vi "ImageDQStagePosition.vi"(11 "Image in":refnum<class "Image.lvclass">) -> (3 "Image out":refnum<class "Image.lvclass">)   [LabVIEW 2012, in "Image.lvclass"]
uses:
  classes/Image.lvclass
  classes/Image.lvclass/Image.ctl
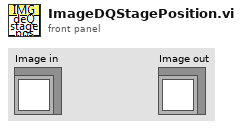
[diagram p1: front panel]
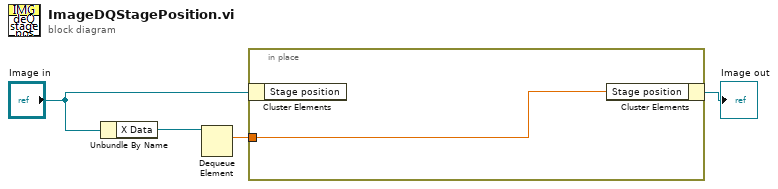
[diagram p0: block diagram]
diagram:
  n1 = Unbundle By Name("Image in") -> ("X Data"=w2:refnum<queue>)
  n2 = Dequeue Element(queue=w2) -> (element=w1:dbl)  [unwired: 2 in, 3 out]
  n3 = in-place {
    in-place-border: w1 -> [w5]
    n4 = in-place-cluster #1("Image in") -> ()  [unwired: 1 out]
    n5 = in-place-cluster #1("Stage position"=w5) -> (→"Image out":refnum<class "Image.lvclass">)
  }
